vi "Balance_PWM.vi"(1 "Balance_Ratio":dbl, 2 "Balance_KD":dbl=-244.0, 3 "Balance_KP":dbl=-50.0, 4 "Angle":dbl) -> (0 "Balance_PWM":dbl)   [LabVIEW 2018]
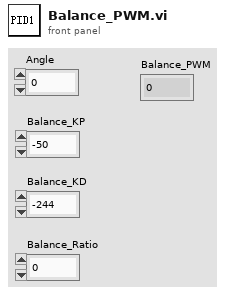
[diagram p1: front panel]
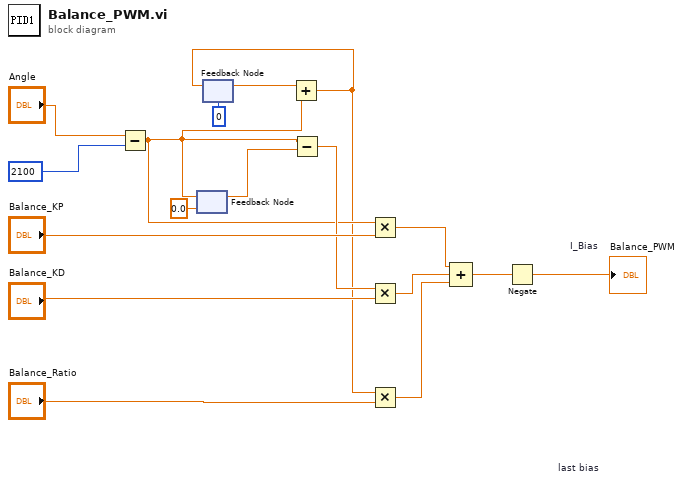
[diagram p0: block diagram]
diagram:
  n1 = Subtract(x="Angle", y=i16 2100) -> (x-y=w7:dbl)
  n2 = feedback-in #1(w7) -> ()
  n3 = feedback #1 "last bias"(0.0) -> (w15:dbl)
  n4 = feedback #2 "I_Bias"(0) -> (w6:dbl)
  n5 = Add(x=w6, y=w7) -> (x+y=w4:dbl)
  n6 = feedback-in #2(w4) -> ()
  n7 = Subtract(x=w7, y=w15) -> (x-y=w13:dbl)
  n8 = Multiply(x=w7, y="Balance_KP") -> (x*y=w11:dbl)
  n9 = Multiply(x=w13, y="Balance_KD") -> (x*y=w10:dbl)
  n10 = Multiply(x=w4, y="Balance_Ratio") -> (x*y=w3:dbl)
  n11 = Compound Arithmetic op=ADD(w11, w10, w3) -> (w2:dbl)
  n12 = Negate(x=w2) -> (-x=→"Balance_PWM":dbl)
